vi "Finish.vi"(0 "Display State In":T1={"Window Handle"=refnum, "Maximum"=100, "State Change Action"=enum."Method - Initialize", "Running"=FALSE, "Visable Items"={"Label"=TRUE, "Caption"=FALSE}, "Value"=100, "Show Progress Bar"=FALSE}, 9 "Container State":T3, 11 "error in (no error)":errorcluster) -> (4 "Display State Out":T1={"Window Handle"=refnum, "Maximum"=100, "State Change Action"=enum."Method - Initialize", "Running"=FALSE, "Visable Items"={"Label"=TRUE, "Caption"=FALSE}, "Value"=100, "Show Progress Bar"=FALSE}, 15 "error out":errorcluster)   [LabVIEW 2011, in "Taskbar Progress Bar.xctl"]
uses:
  Taskbar Progress Bar.xctl
  <vilib>/_xctls/Container State.ctl
  Abilities/TPB State.ctl
  TypeDefs/Dispaly State Change Methods.ctl
  <vilib>/_xctls/XControlSupport.lvlib
panel:
  # "Add Controls & Indicators that form the parameters of the method here. Hook them to the connector pane. Do not delete the controls & indicators that are already hooked to the connector pane.\n \nTo setup the parameters  for this method, right click on this item in the Project Tree & select \"Configure Method...\"."
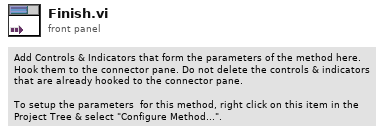
[diagram p1: front panel]
types:
  T1 = typedef "Taskbar Progress Bar.xctl/TPB State.ctl" = cluster{"Window Handle":refnum<k24>, "Maximum":u64, "State Change Action":T2, "Running":bool, "Visable Items":cluster{"Label":bool, "Caption":bool}, "Value":u64, "Show Progress Bar":bool}
  T2 = typedef "Taskbar Progress Bar.xctl/Dispaly State Change Methods.ctl" = enum16{"No Action", "Created", "Method - Initialize", "Method - Increment", "Method - Set Value", "Method - Pause", "Method - Error", "Method - Finish", "Property - Show Progress Bar"}
  T3 = typedef "XControlSupport.lvlib/Container State.ctl" = cluster{"Indicator?":bool, "Run Mode?":bool, " Refnum":refnum<vi>}
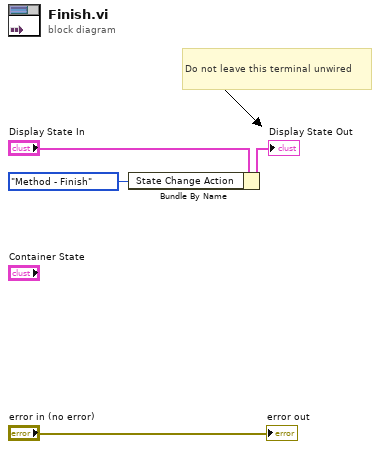
[diagram p0: block diagram]
diagram:
  # "Do not leave this terminal unwired"
  n1 = Bundle By Name(cluster="Display State In", "State Change Action"=Dispaly_State_Change_Methods."Method - Finish") -> (→"Display State Out":T1)
  "error out" <- "error in (no error)"
